vi "VisionX-2LOOPs-Main.vi"() -> ()   [LabVIEW 2020]
uses:
  <vilib>/vision/Measure.llb/Straight Edge Options.ctl
  <vilib>/vision/Measure.llb/Straight Edge Process.ctl
  _FW/Cmd.ctl
  _FW/TestState.ctl
  <vilib>/vision/Image Controls.llb/IMAQ Image.ctl
  <vilib>/vision/Measure.llb/Edge Options.ctl
  <vilib>/vision/Measure.llb/Edge Polarity.ctl
  <vilib>/vision/NI_Vision_Development_Module.lvlib
panel:
  out "Image":T1(plugin-control)
  in  "Line Fit Options":T2={"Number of Lines"=1, "Type"=enum."Best Edge Rake", "Min. Score"=10.0, "Max. Score"=1000.0, "Orientation"=0.0, "Angle Range"=45.0, "Angle Tolerance"=1.0, "Step Size"=7, "Min. SNR (db)"=0.0, "Min. Points (%)"=25.0, "Hough Iterations"=5} {"Min. Points (%)" min=0.0 max=100.0; "Min. SNR (db)" min=0.0; "Max. Score" min=0.0 max=1024.0; "Min. Score" min=0.0 max=1024.0 step=1.0}
  out "Liquied Level":dbl format="%.2f"
  out "Pass?":bool
  in  "PauseTest":bool
  in  "StartTest":bool
  out "ErrO":errorcluster
  in  "ErrI":errorcluster
  in  "Exit":bool
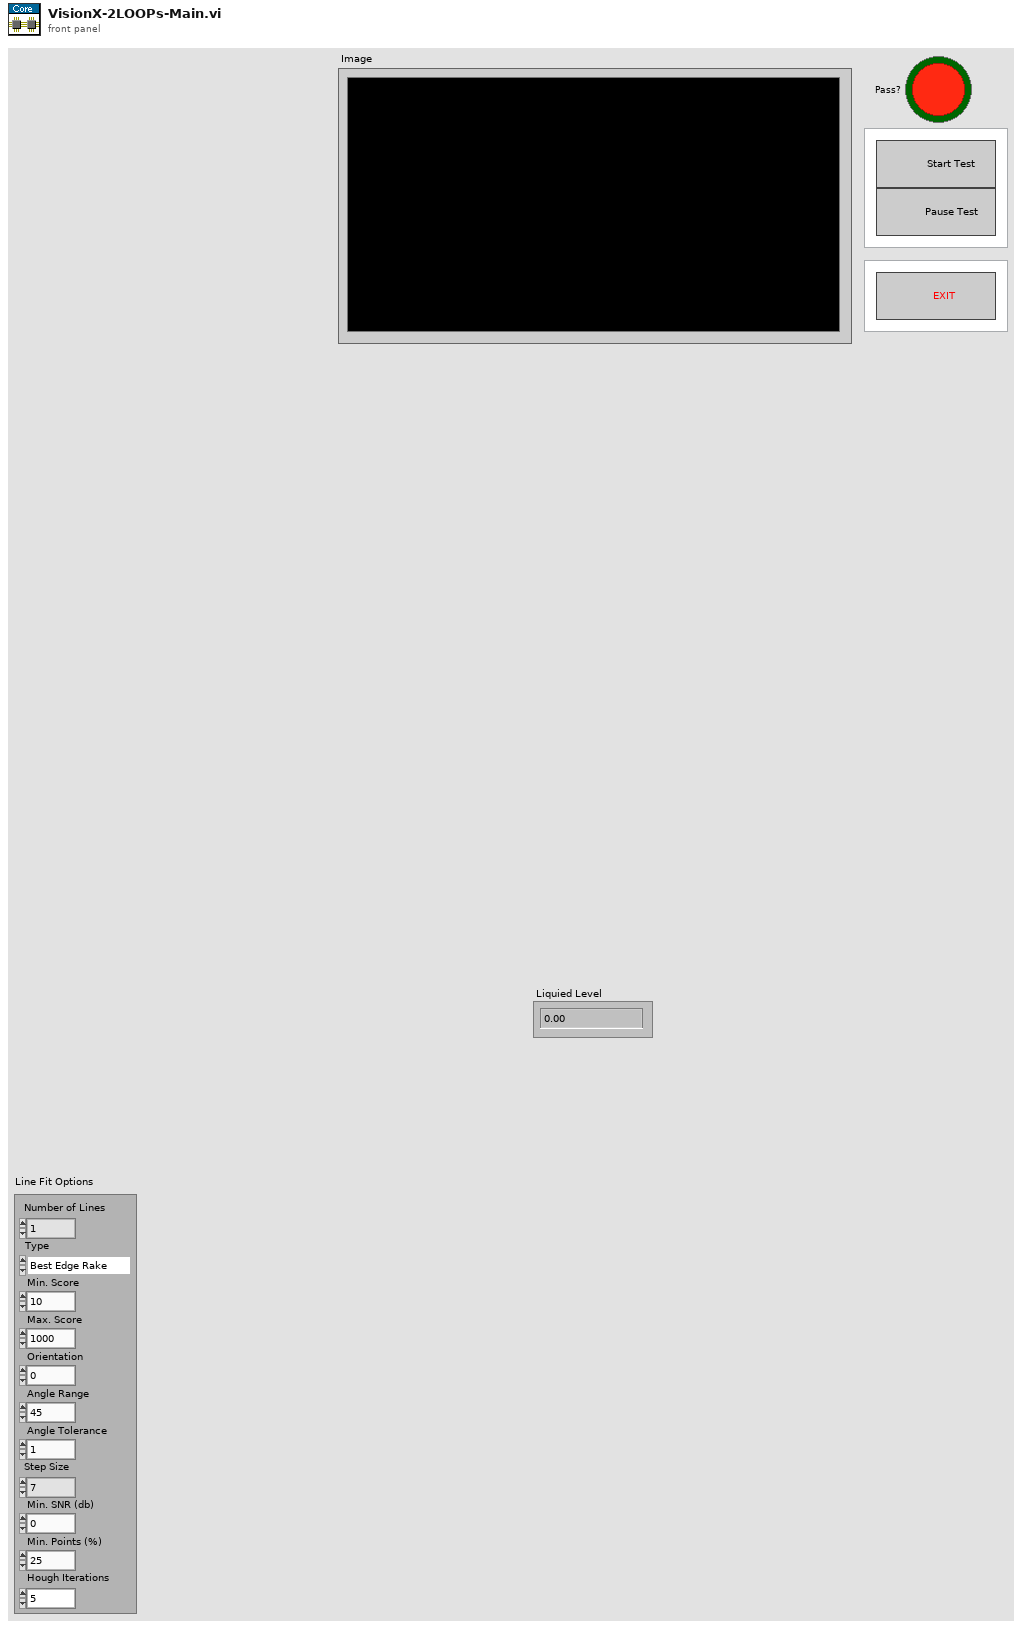
[diagram p1: front panel]
types:
  T1 = typedef "IMAQ Image.ctl" = refnum<image>
  T2 = typedef "Straight Edge Options.ctl" = cluster{"Number of Lines":i32, "Type":T3, "Min. Score":dbl, "Max. Score":dbl, "Orientation":dbl, "Angle Range":dbl, "Angle Tolerance":dbl, "Step Size":u32, "Min. SNR (db)":dbl, "Min. Points (%)":dbl, "Hough Iterations":i32}
  T3 = typedef "Straight Edge Process.ctl" = enum32{"First Edge Rake", "Best Edge Rake", "Hough Edge Rake", "First Edge Projection", "Best Edge Projection"}
  T4 = typedef "Cmd.ctl" = enum16{"idle", "---------- APP ---------", "APP::Init", "APP::Exit", "-------- ERROR --------", "ERR::Handler", "------ TEST PLAN ------", "TEST::Prep", "TEST::Start", "TEST::Run", "TEST::Pause", "TEST::Exit", "---- MACHINE VISION----", "MV::Init", "MV::Prep", "MV::SetROI", "MV::Cord", "MV::Check", "MV::Clean", "--------- USER ----------", "USER::Case1", "USER::Case2"}
  T5 = typedef "TestState.ctl" = enum16{"Idle", "Running"}
  T6 = typedef "IMAQ Rectangle" = cluster{"Left":i32, "Top":i32, "Right":i32, "Bottom":i32, "Rotation":dbl}
  T7 = cluster{"Point1":cluster{"X":sgl, "Y":sgl}, "Point2":cluster{"X":sgl, "Y":sgl}}
  T8 = typedef "IMAQ Coordinate System" = cluster{"Reference System":cluster{"Origin":cluster{"X":sgl, "Y":sgl}, "Angle (deg)":sgl, "Axis Reference":u32}, "Measurement System":cluster{"Origin":cluster{"X":sgl, "Y":sgl}, "Angle (deg)":sgl, "Axis Reference":u32}}
  T9 = cluster{"Src":T1, "Dst":T1, "Parts":string[], "RefCoord":T8, "MsrCoord":T8, "MsrROI":T6, "RefLine":cluster{"Point1":cluster{"X":sgl, "Y":sgl}, "Point2":cluster{"X":sgl, "Y":sgl}}}
  T10 = typedef "Edge Options.ctl" = cluster{"Edge Polarity":T11, "Kernel Size":u32, "Width":u32, "Minimum Edge Strength":sgl, "Interpolation Type":enum32{"Zero Order", "Bilinear", "Quadratic", "Cubic", "Bilinear Fixed"}, "Data Processing Method":enum32{"Average", "Median"}}
  T11 = typedef "Edge Polarity.ctl" = u32
  T12 = cluster{"Direction":u16, "Primary Edge Options":T10, "Secondary Edge Options":T10, "Show Search Area":bool, "Show Search Lines":bool, "Show Edges Found":bool, "Show Result":bool, "Search Area Color":u32, "Search Lines Color":u32, "Edge Locations Color":u32, "Result Color":u32, "Overlay Group Name":string}
  T13 = typedef "ROI Descriptor" = cluster{"Global Rectangle":i32[], "Contours":cluster{"ID":enum32{"External", "Internal"}, "Type":u32, "Coordinates":i32[]}[]}
  T14 = cluster{"Search Direction":u32, "Edge Options":T10, "Show Search Area":bool, "Show Search Lines":bool, "Show Edges Found":bool, "Show Result":bool, "Search Area Color":u32, "Search Lines Color":u32, "Edge Locations Color":u32, "Result Color":u32, "Overlay Group Name":string}
  T15 = cluster{"Point1 (Pixels)":cluster{"X":sgl, "Y":sgl}, "Point2 (Pixels)":cluster{"X":sgl, "Y":sgl}, "Point1 (Real-World)":cluster{"X":sgl, "Y":sgl}, "Point2 (Real-World)":cluster{"X":sgl, "Y":sgl}, "Angle (Pixel)":dbl, "Angle (Real-World)":dbl, "Score":dbl, "Straightness":dbl, "Average SNR (db)":dbl, "Calibration Valid":bool}[]
  T16 = cluster{"Point1 (Pixels)":cluster{"X":sgl, "Y":sgl}, "Point2 (Pixels)":cluster{"X":sgl, "Y":sgl}, "Point1 (Real-World)":cluster{"X":sgl, "Y":sgl}, "Point2 (Real-World)":cluster{"X":sgl, "Y":sgl}, "Angle (Pixel)":dbl, "Angle (Real-World)":dbl, "Score":dbl, "Straightness":dbl, "Average SNR (db)":dbl, "Calibration Valid":bool}
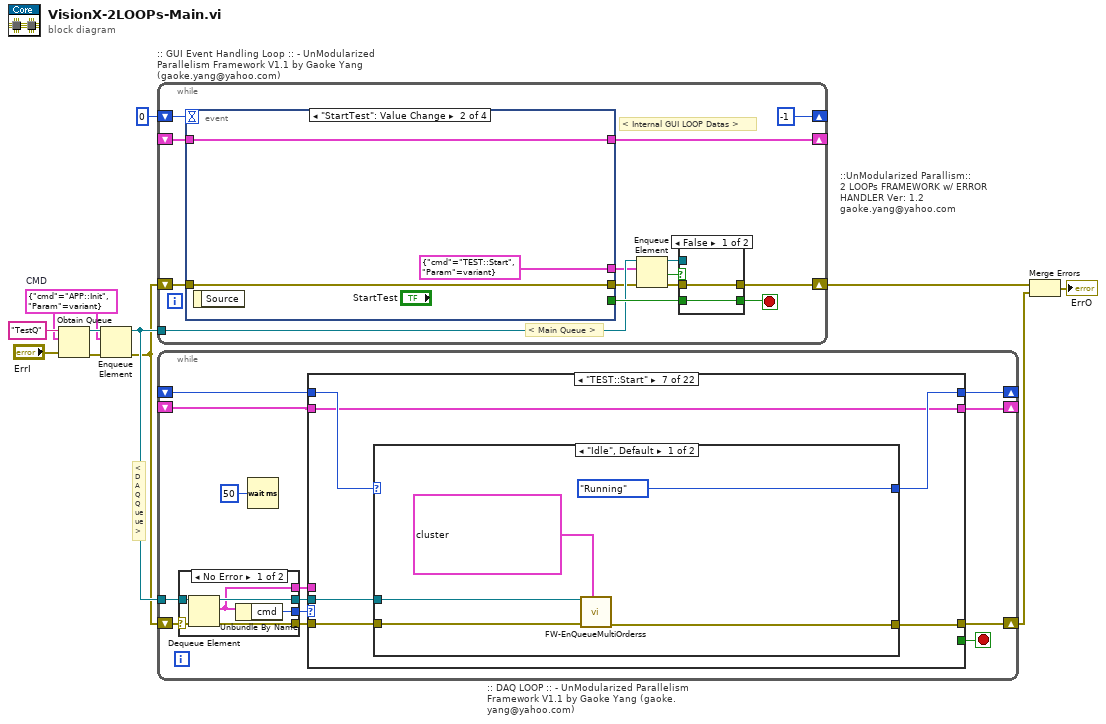
[diagram p0: block diagram]
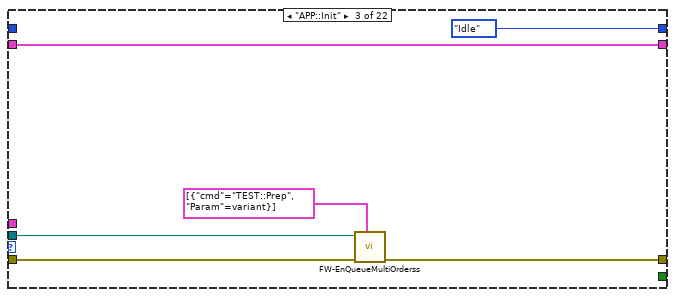
[diagram p4: hidden frame]
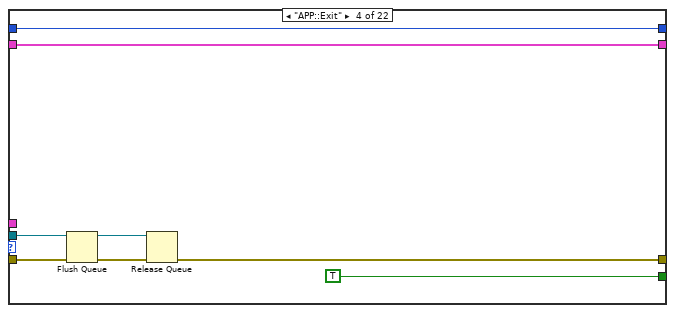
[diagram p5: hidden frame]
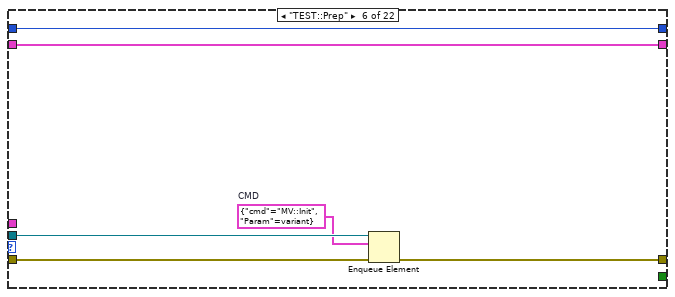
[diagram p7: hidden frame]
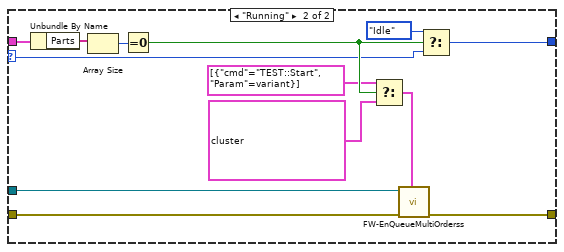
[diagram p10: hidden frame]
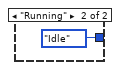
[diagram p12: hidden frame]
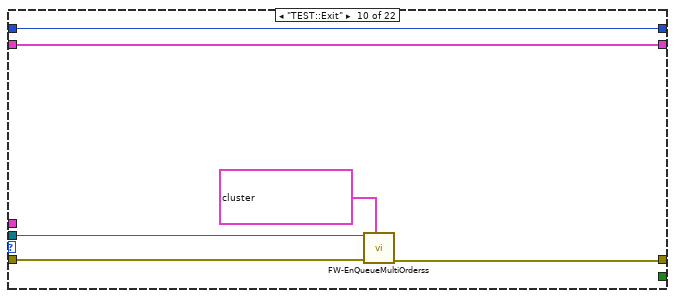
[diagram p13: hidden frame]
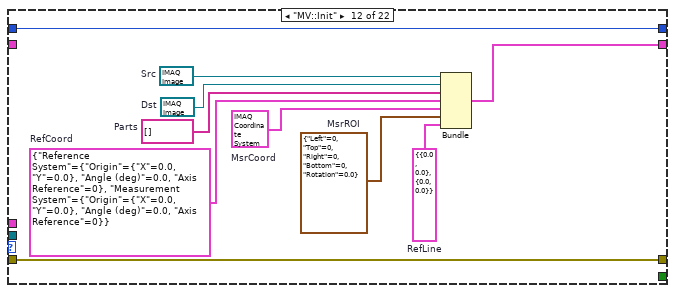
[diagram p15: hidden frame]
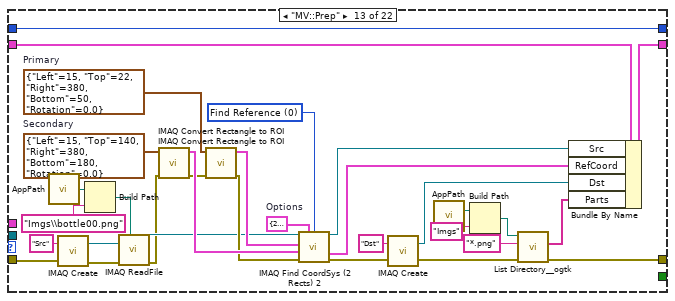
[diagram p16: hidden frame]
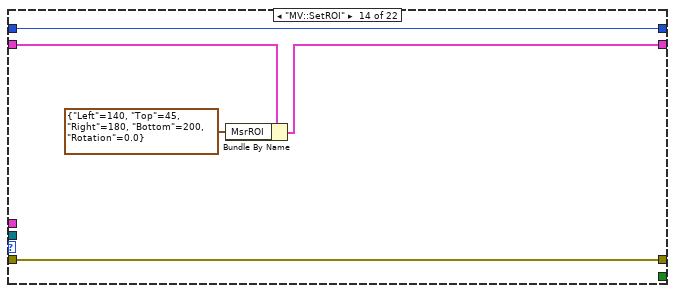
[diagram p17: hidden frame]
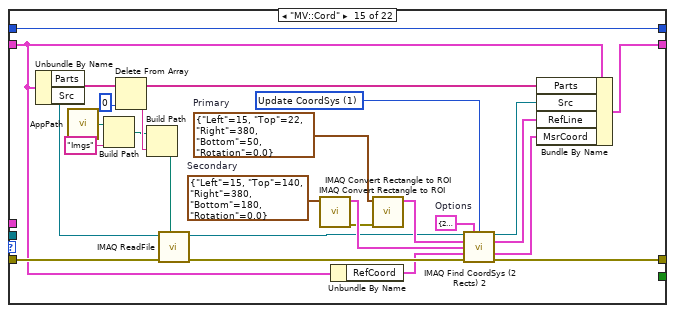
[diagram p18: hidden frame]
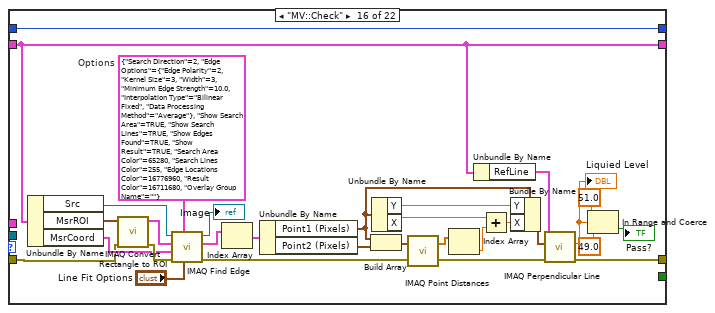
[diagram p19: hidden frame]
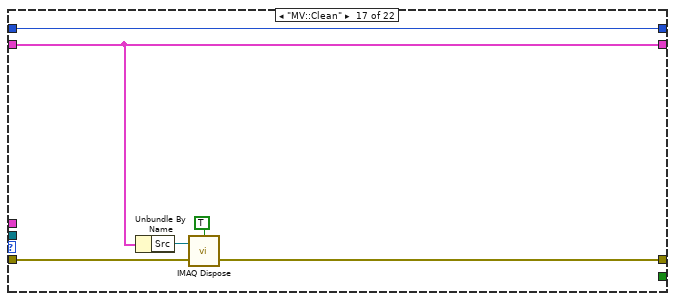
[diagram p20: hidden frame]
diagram:
  w2 = cluster{"cmd":T4, "Param":variant} {"cmd"=enum."APP::Init", "Param"=variant}  # CMD
  # "::UnModularized Parallism::\n2 LOOPs FRAMEWORK w/ ERROR HANDLER Ver: 1.2\ngaoke.yang@yahoo.com"
  # "< DAQ Queue >"
  n1 = Obtain Queue(name (unnamed)="TestQ", element data type=w2, error in (no error)="ErrI") -> (queue out=w10:refnum<queue>, error out=w9:errorcluster)  [unwired: 2 in, 1 out]
  n2 = Enqueue Element(queue=w10, element=w2, error in (no error)=w9) -> (queue out=w7:refnum<queue>, error out=w6:errorcluster)  [unwired: 2 out]
  n3 = while ":: GUI Event Handling Loop :: - UnModularized Parallelism Framework V1.1 by Gaoke Yang (gaoke.yang@yahoo.com)" {
    tunnel: w7 -> [w15]
    shift-right: [w24] -> w11
    shift-left: w6 -> [w25]
    shift-right: [-1] -> _
    shift-left: 0 -> [w22]
    shift-right: [w21] -> _
    shift-left: _ -> [w20]
    stop <- w18 stop-if-true
    # "< Internal GUI LOOP Datas >"
    # "< Main Queue >"
    n4 = event shown="[1] \"StartTest\": Value Change" {
      selector: _ -> [_ _ _ _]
      dyn-events: _ -> [_ _ _ _]
      timeout: w22 -> [_ _ _ _]
      tunnel: [_ _ _ TRUE ("Exit")] -> w19
      tunnel: w25 -> [w34 w37 w39 w41]
      tunnel: [w34 w37 w39 w41] -> w14
      tunnel: [_ cluster{"cmd":T4, "Param":variant} {"cmd"=enum."TEST::Start", "Param"=variant} ("CMD") cluster{"cmd":T4, "Param":variant} {"cmd"=enum."TEST::Pause", "Param"=variant} ("CMD") cluster{"cmd":T4, "Param":variant} {"cmd"=enum."TEST::Exit", "Param"=variant} ("CMD")] -> w13
      tunnel: [w32 w36 _ w43] -> w21
      tunnel: w20 -> [_ w36 _ w43]
      event Timeout {
        w33 = FALSE  # GUI Data Example
        # "Timeout:\n- This Case will only bee excuted for 1 time since timeout=0;\nNotes:\n- Used this place as a GUI Initializer."
        n5 = event-data() -> ()  [unwired: 2 out]
        n6 = Bundle("GUI Data Example"=w33) -> (w32:cluster{"GUI Data Example":bool})  [unwired: 1 in]
      }
      event "StartTest": Value Change {
        n7 = event-data() -> ()  [unwired: 2 out]
      }
      event "PauseTest": Value Change {
        # "PauseDQA  Button clicked\n- Send Pause DAQ command to start the DAQ.\nNotes:"
        n8 = event-data() -> ()  [unwired: 2 out]
      }
      event "Exit": Value Change; Panel Close {
        # "Exit Button clicked or panel was closed\n- Send Exit commands and Exit Application\nNotes:"
        n9 = event-data() -> ()  [unwired: 2 out]
      }
    }
    n10 = Enqueue Element(queue=w15, element=w13, error in (no error)=w14) -> (queue out=w17:refnum<queue>, timed out?=w16:bool, error out=w12:errorcluster)  [unwired: 1 out]
    n11 = case shown="False" w16 {
      tunnel: [w26 w29] -> w24
      tunnel: w19 -> [w27 _]
      tunnel: [w27 TRUE ("Exit")] -> w18
      tunnel: w17 -> [_ w30]
      tunnel: w12 -> [w26 w28]
      frame False {
      }
      frame True {
        n12 = Release Queue(queue=w30, error in (no error)=w28) -> (error out=w29:errorcluster)  [unwired: 1 in, 2 out]
      }
    }
  }
  n13 = while ":: DAQ LOOP :: - UnModularized Parallelism Framework V1.1 by Gaoke Yang (gaoke.yang@yahoo.com)" {
    tunnel: w7 -> [w56]
    shift-right: [w49] -> w5
    shift-left: w6 -> [w55]
    shift-right: [w47] -> _
    shift-left: _ -> [w54]
    shift-right: [w46] -> _
    shift-left: _ -> [w45]
    stop <- w48 stop-if-true
    n14 = case shown="No Error" w55 {
      selector: w55 -> [w270 w276]
      tunnel: w56 -> [w273 w275]
      tunnel: [w272 w276] -> w53
      tunnel: [w271 w275] -> w50
      tunnel: [w268 Cmd."ERR::Handler" ("Enum")] -> w52
      tunnel: [w269 _] -> w51
      frame No Error {
        n15 = Dequeue Element(queue=w273, error in (no error)=w270) -> (queue out=w271:refnum<queue>, element=w269:cluster{"cmd":T4, "Param":variant}, error out=w272:errorcluster)  [unwired: 2 out]
        n16 = Unbundle By Name(w269) -> ("cmd"=w268:T4)
      }
      frame Error {
      }
    }
    n17 = Wait (ms)(milliseconds to wait=u32 50) -> ()  [unwired: 1 out]
    n18 = case shown="\"TEST::Start\"" w52 {
      tunnel: [w59 w61 w65 w71 w79 w82 w90 w102 w122 w129 w134 w136 w170 w178 w192 w217 w244 w247 w251 w260 w263 w266] -> w49
      tunnel: [_ _ _ TRUE _ _ _ _ _ _ _ _ _ _ _ _ _ _ w250 _ _ _] -> w48
      tunnel: [w58 w62 w68 w75 w78 w85 w86 w99 w123 w127 w133 w144 w174 w181 w204 w216 w243 w246 w252 w261 w264 w267] -> w47
      tunnel: w54 -> [w58 w62 w68 w75 w78 w85 w86 w99 w123 w127 w133 _ w175 w180 w184 w216 w243 w246 w253 w261 w264 w267]
      tunnel: w53 -> [w59 w61 w66 w70 w79 w83 w91 w103 w122 w130 w134 w136 w146 w178 w185 w210 w240 w247 w249 w260 w263 w266]
      tunnel: w51 -> [_ _ _ _ _ _ _ _ _ _ _ _ _ _ _ _ _ _ _ _ _ _]
      tunnel: w50 -> [_ _ w67 w72 _ w81 w87 w104 _ w128 _ _ _ _ _ _ _ _ _ _ _ _]
      tunnel: [w57 w60 TestState."Idle" ("TestState") w69 w77 w84 w88 w100 w121 w126 w132 w135 w145 w177 w182 w209 w239 w245 w248 w259 w262 w265] -> w46
      tunnel: w45 -> [w57 w60 _ w69 w77 w84 w89 w101 w120 w126 w132 w135 w145 w177 w182 w209 w239 w245 w248 w259 w262 w265]
      frame "idle" {
      }
      frame "---------- APP ---------" {
      }
      frame "APP::Init" {
        n19 = call "FW-EnQueueMultiOrderss.vi"("CMDs"=cluster{"cmd":T4, "Param":variant}[] [{"cmd"=enum."TEST::Prep", "Param"=variant}], "ErrorIn"=w66, "QueueIn"=w67) -> ("ErrorOut"=w65:errorcluster)  [unwired: 7 in, 1 out]
      }
      frame "APP::Exit" {
        n20 = Flush Queue(queue=w72, error in (no error)=w70) -> (queue out=w74:refnum<queue>, error out=w73:errorcluster)  [unwired: 1 out]
        n21 = Release Queue(queue=w74, error in (no error)=w73) -> (error out=w71:errorcluster)  [unwired: 1 in, 2 out]
      }
      frame "------ TEST PLAN ------" {
      }
      frame "TEST::Prep" {
        w80 = cluster{"cmd":T4, "Param":variant} {"cmd"=enum."MV::Init", "Param"=variant}  # CMD
        n22 = Enqueue Element(queue=w81, element=w80, error in (no error)=w83) -> (error out=w82:errorcluster)  [unwired: 3 out]
      }
      frame "TEST::Start" {
        n23 = case shown="\"Idle\", Default" w89 {
          selector: w89 -> [_ w97]
          tunnel: [w92 w98] -> w90
          tunnel: w91 -> [w96 w98]
          tunnel: [TestState."Running" ("TestState") w97] -> w88
          tunnel: w87 -> [w94 _]
          frame "Idle", Default {
            n24 = call "FW-EnQueueMultiOrderss.vi"("CMDs"=cluster{"cmd":T4, "Param":variant}[] [{"cmd"=enum."MV::Prep", "Param"=variant}, {"cmd"=enum."MV::SetROI", "Param"=variant}, {"cmd"=enum."TEST::Run", "Param"=variant}], "ErrorIn"=w96, "QueueIn"=w94) -> ("ErrorOut"=w92:errorcluster)  [unwired: 7 in, 1 out]
          }
          frame "Running" {
          }
        }
      }
      frame "TEST::Run" {
        n25 = case shown="\"Idle\", Default" w101 {
          selector: w101 -> [w106 w111]
          tunnel: w104 -> [_ w119]
          tunnel: w103 -> [w105 w118]
          tunnel: [w105 w110] -> w102
          tunnel: [w106 w112] -> w100
          tunnel: w99 -> [_ w115]
          frame "Idle", Default {
          }
          frame "Running" {
            n26 = Unbundle By Name(w115) -> ("Parts"=w117:string[])
            n27 = Array Size(array=w117) -> (size(s)=w116:i32)
            n28 = Equal To 0?(x=w116) -> (x = 0?=w114:bool)
            n29 = Select(t=cluster{"cmd":T4, "Param":variant}[] [{"cmd"=enum."TEST::Start", "Param"=variant}], s=w114, f=cluster{"cmd":T4, "Param":variant}[] [{"cmd"=enum."MV::Cord", "Param"=variant}, {"cmd"=enum."MV::Check", "Param"=variant}, {"cmd"=enum."TEST::Run", "Param"=variant}]) -> (s? t:f=w107:cluster{"cmd":T4, "Param":variant}[])
            n30 = call "FW-EnQueueMultiOrderss.vi"("CMDs"=w107, "ErrorIn"=w118, "QueueIn"=w119) -> ("ErrorOut"=w110:errorcluster)  [unwired: 7 in, 1 out]
            n31 = Select(t=TestState."Idle" ("TestState"), s=w114, f=w111) -> (s? t:f=w112:T5)
          }
        }
      }
      frame "TEST::Pause" {
        n32 = case shown="\"Idle\", Default" w120 {
          selector: w120 -> [w124 _]
          tunnel: [w124 TestState."Idle" ("TestState")] -> w121
          frame "Idle", Default {
          }
          frame "Running" {
          }
        }
      }
      frame "TEST::Exit" {
        n33 = call "FW-EnQueueMultiOrderss.vi"("CMDs"=cluster{"cmd":T4, "Param":variant}[] [{"cmd"=enum."MV::Clean", "Param"=variant}, {"cmd"=enum."APP::Exit", "Param"=variant}], "ErrorIn"=w130, "QueueIn"=w128) -> ("ErrorOut"=w129:errorcluster)  [unwired: 7 in, 1 out]
      }
      frame "---- MACHINE VISION----" {
      }
      frame "MV::Init" {
        w137 = T7 {"Point1"={"X"=0.0, "Y"=0.0}, "Point2"={"X"=0.0, "Y"=0.0}}  # RefLine
        w138 = T6 {"Left"=0, "Top"=0, "Right"=0, "Bottom"=0, "Rotation"=0.0}  # MsrROI
        w139 = T8 {"Reference System"={"Origin"={"X"=0.0, "Y"=0.0}, "Angle (deg)"=0.0, "Axis Reference"=0}, "Measurement System"={"Origin"={"X"=0.0, "Y"=0.0}, "Angle (deg)"=0.0, "Axis Reference"=0}}  # MsrCoord
        w140 = T8 {"Reference System"={"Origin"={"X"=0.0, "Y"=0.0}, "Angle (deg)"=0.0, "Axis Reference"=0}, "Measurement System"={"Origin"={"X"=0.0, "Y"=0.0}, "Angle (deg)"=0.0, "Axis Reference"=0}}  # RefCoord
        w143 = T1 refnum  # Dst
        w142 = string[] []  # Parts
        w141 = T1 refnum  # Src
        n34 = Bundle("Src"=w141, "Dst"=w143, "Parts"=w142, "RefCoord"=w140, "MsrCoord"=w139, "MsrROI"=w138, "RefLine"=w137) -> (w144:T9)  [unwired: 1 in]
      }
      frame "MV::Prep" {
        w162 = T6 {"Left"=15, "Top"=140, "Right"=380, "Bottom"=180, "Rotation"=0.0}  # Secondary
        w163 = T6 {"Left"=15, "Top"=22, "Right"=380, "Bottom"=50, "Rotation"=0.0}  # Primary
        w161 = T12 {"Direction"=2, "Primary Edge Options"={"Edge Polarity"=0, "Kernel Size"=3, "Width"=3, "Minimum Edge Strength"=10.0, "Interpolation Type"=enum."Bilinear Fixed", "Data Processing Method"=enum."Average"}, "Secondary Edge Options"={"Edge Polarity"=0, "Kernel Size"=3, "Width"=3, "Minimum Edge Strength"=10.0, "Interpolation Type"=enum."Bilinear Fixed", "Data Processing Method"=enum."Average"}, "Show Search Area"=TRUE, "Show Search Lines"=TRUE, "Show Edges Found"=TRUE, "Show Result"=TRUE, "Search Area Color"=65280, "Search Lines Color"=255, "Edge Locations Color"=14811391, "Result Color"=16711704, "Overlay Group Name"=""}  # Options
        w165 = u16 0 items=["Find Reference", "Update CoordSys"] ("Mode")
        n35 = call "AppPath.vi"() -> ("AppPath"=w152:path)
        n36 = call "IMAQ Create"("Image Name"="Src", "error in (no error)"=w146) -> ("New Image"=w173:T1, "error out"=w172:errorcluster)  [unwired: 3 in]
        n37 = Build Path(base path=w152, name or relative path="Imgs\\bottle00.png") -> (appended path=w150:path)
        n38 = call "IMAQ ReadFile"("File Path"=w150, "error in (no error)"=w172, "Image"=w173) -> ("error out"=w156:errorcluster, "Image Out"=w157:T1)  [unwired: 4 in, 3 out]
        n39 = call "IMAQ Convert Rectangle to ROI"("error in (no error)"=w156, "Rectangle"=w162) -> ("error out"=w160:errorcluster, "ROI Descriptor"=w164:T13)  [unwired: 7 in]
        n40 = call "IMAQ Convert Rectangle to ROI"("error in (no error)"=w160, "Rectangle"=w163) -> ("error out"=w159:errorcluster, "ROI Descriptor"=w158:T13)  [unwired: 7 in]
        n41 = call "IMAQ Find CoordSys (2 Rects) 2"("Image"=w157, "Options"=w161, "Mode"=w165, "Primary ROI Descriptor"=w158, "Secondary ROI Descriptor"=w164, "error in (no error)"=w159) -> ("Image Out"=w154:T1, "Coordinate System Out"=w153:T8, "error out"=w155:errorcluster)  [unwired: 5 in, 2 out]
        n42 = call "IMAQ Create"("Image Name"="Dst", "error in (no error)"=w155) -> ("New Image"=w167:T1, "error out"=w168:errorcluster)  [unwired: 3 in]
        n43 = call "AppPath.vi"() -> ("AppPath"=w148:path)
        n44 = Build Path(base path=w148, name or relative path="Imgs") -> (appended path=w147:path)
        n45 = call "List Directory__ogtk.vi"("error in (no error)"=w168, "pattern"="*.png", "directory path"=w147) -> ("error out"=w170:errorcluster, "file names"=w166:string[])  [unwired: 1 in, 2 out]
        n46 = Bundle By Name(cluster=w175, "Src"=w154, "RefCoord"=w153, "Dst"=w167, "Parts"=w166) -> (w174:T9)
      }
      frame "MV::SetROI" {
        n47 = Bundle By Name(cluster=w180, "MsrROI"=T6 {"Left"=140, "Top"=45, "Right"=180, "Bottom"=200, "Rotation"=0.0} ("Rectangle")) -> (w181:T9)
      }
      frame "MV::Cord" {
        w198 = T6 {"Left"=15, "Top"=140, "Right"=380, "Bottom"=180, "Rotation"=0.0}  # Secondary
        w199 = T6 {"Left"=15, "Top"=22, "Right"=380, "Bottom"=50, "Rotation"=0.0}  # Primary
        w197 = T12 {"Direction"=2, "Primary Edge Options"={"Edge Polarity"=0, "Kernel Size"=3, "Width"=3, "Minimum Edge Strength"=10.0, "Interpolation Type"=enum."Bilinear Fixed", "Data Processing Method"=enum."Average"}, "Secondary Edge Options"={"Edge Polarity"=0, "Kernel Size"=3, "Width"=3, "Minimum Edge Strength"=10.0, "Interpolation Type"=enum."Bilinear Fixed", "Data Processing Method"=enum."Average"}, "Show Search Area"=TRUE, "Show Search Lines"=TRUE, "Show Edges Found"=TRUE, "Show Result"=TRUE, "Search Area Color"=65280, "Search Lines Color"=255, "Edge Locations Color"=14811391, "Result Color"=16711704, "Overlay Group Name"=""}  # Options
        w201 = u16 1 items=["Find Reference", "Update CoordSys"] ("Mode")
        n48 = Unbundle By Name(w184) -> ("Parts"=w203:string[], "Src"=w202:T1)
        n49 = call "AppPath.vi"() -> ("AppPath"=w188:path)
        n50 = Build Path(base path=w188, name or relative path="Imgs") -> (appended path=w187:path)
        n51 = Delete From Array(array=w203, index=0) -> (deleted portion=w207:string, array with subset deleted=w205:string[])  [unwired: 1 in]
        n52 = Build Path(base path=w187, name or relative path=w207) -> (appended path=w206:path)
        n53 = call "IMAQ ReadFile"("File Path"=w206, "error in (no error)"=w185, "Image"=w202) -> ("error out"=w194:errorcluster, "Image Out"=w193:T1)  [unwired: 4 in, 3 out]
        n54 = call "IMAQ Convert Rectangle to ROI"("Rectangle"=w198) -> ("error out"=w196:errorcluster, "ROI Descriptor"=w200:T13)  [unwired: 8 in]
        n55 = Unbundle By Name(w184) -> ("RefCoord"=w183:T8)
        n56 = call "IMAQ Convert Rectangle to ROI"("error in (no error)"=w196, "Rectangle"=w199) -> ("ROI Descriptor"=w195:T13)  [unwired: 7 in, 1 out]
        n57 = call "IMAQ Find CoordSys (2 Rects) 2"("Image"=w193, "Options"=w197, "Mode"=w201, "Primary ROI Descriptor"=w195, "Secondary ROI Descriptor"=w200, "Coordinate System In"=w183, "error in (no error)"=w194) -> ("Image Out"=w191:T1, "Main Axis"=w190:T7, "Coordinate System Out"=w189:T8, "error out"=w192:errorcluster)  [unwired: 4 in, 1 out]
        n58 = Bundle By Name(cluster=w184, "Parts"=w205, "Src"=w191, "RefLine"=w190, "MsrCoord"=w189) -> (w204:T9)
      }
      frame "MV::Check" {
        w232 = T14 {"Search Direction"=2, "Edge Options"={"Edge Polarity"=2, "Kernel Size"=3, "Width"=3, "Minimum Edge Strength"=10.0, "Interpolation Type"=enum."Bilinear Fixed", "Data Processing Method"=enum."Average"}, "Show Search Area"=TRUE, "Show Search Lines"=TRUE, "Show Edges Found"=TRUE, "Show Result"=TRUE, "Search Area Color"=65280, "Search Lines Color"=255, "Edge Locations Color"=16776960, "Result Color"=16711680, "Overlay Group Name"=""}  # Options
        n59 = Unbundle By Name(w216) -> ("Src"=w238:T1, "MsrROI"=w236:T6, "MsrCoord"=w234:T8)
        n60 = call "IMAQ Convert Rectangle to ROI"("error in (no error)"=w210, "Rectangle"=w236) -> ("error out"=w237:errorcluster, "ROI Descriptor"=w235:T13)  [unwired: 7 in]
        n61 = call "IMAQ Find Edge"("Line Fit Options"="Line Fit Options", "Options"=w232, "error in (no error)"=w237, "Coordinate System"=w234, "ROI Descriptor"=w235, "Image"=w238) -> ("error out"=w227:errorcluster, "Straight Edges"=w230:T15, "Image Out"=→"Image":T1)  [unwired: 2 in, 1 out]
        n62 = Index Array(array=w230) -> (element=w229:T16)  [unwired: 1 in]
        n63 = Unbundle By Name(w229) -> ("Point1 (Pixels)"=w220:cluster{"X":sgl, "Y":sgl}, "Point2 (Pixels)"=w219:cluster{"X":sgl, "Y":sgl})
        n64 = Build Array(w220, w219) -> (w228:cluster{"X":sgl, "Y":sgl}[])
        n65 = Unbundle By Name(w220) -> ("Y"=w223:sgl, "X"=w226:sgl)
        n66 = call "IMAQ Point Distances"("Points"=w228, "error in (no error)"=w227) -> ("Distances"=w225:sgl[], "error out"=w218:errorcluster)  [unwired: 3 in]
        n67 = Index Array(array=w225) -> (element=w224:sgl)  [unwired: 1 in]
        n68 = Unbundle By Name(w216) -> ("RefLine"=w215:T7)
        n69 = Add(x=w226, y=w224) -> (x+y=w222:sgl)
        n70 = Bundle By Name(cluster=w220, "Y"=w223, "X"=w222) -> (w221:cluster{"X":sgl, "Y":sgl})
        n71 = call "IMAQ Perpendicular Line"("error in (no error)"=w218, "Point"=w221, "Line"=w215) -> ("error out"=w217:errorcluster, "Distance"=w214:dbl)  [unwired: 6 in, 1 out]
        "Liquied Level" <- w214
        n72 = In Range and Coerce(upper limit=51.0, x=w214, lower limit=49.0) -> (In Range?=→"Pass?":bool)  [unwired: 1 out]
      }
      frame "MV::Clean" {
        n73 = Unbundle By Name(w243) -> ("Src"=w242:T1)
        n74 = call "IMAQ Dispose"("All Images? (No)"=TRUE, "Image"=w242, "error in (no error)"=w240) -> ("error out"=w244:errorcluster)  [unwired: 3 in]
      }
      frame "-------- ERROR --------" {
      }
      frame "ERR::Handler" {
        n75 = Unbundle By Name(w249) -> ("code"=w254:i32)
        n76 = case shown="0, Default" w254 {
          tunnel: [w258] -> w252
          tunnel: w253 -> [w258]
          tunnel: [errorcluster {"status"=FALSE, "code"=0, "source"=""} ("error out")] -> w251
          tunnel: [TRUE] -> w250
          tunnel: w249 -> [w256]
          frame 0, Default {
            # "Default Error Code Handling Case\n- Report Error\n- Clear Error \nNotes:\n- Add error handling case if you want to handle specific error code."
            n77 = call <vilib>:"General Error Handler.vi"("error in (no error)"=w256) -> ()  [unwired: 10 in, 5 out]
          }
        }
      }
      frame "--------- USER ----------" {
      }
      frame "USER::Case1" {
      }
      frame "USER::Case2" {
      }
    }
  }
  n78 = Merge Errors(w11, w5) -> (→"ErrO":errorcluster)
